vi "CanTest.vi"() -> ()   [LabVIEW 2015]
uses:
  Crl/Can_DataType.ctl
panel:
  in  "SCUBoot":bool
  out "RespGood？":bool
  in  "Clear":bool
  in  "Seq?":bool
  in  "EXIT":bool
  in  "identifier":u32=1238 format="%x"
  in  "select？":bool
  in  "Send Data":T1=[{"identifier"=1715, "payload"=[3, 34, 241, 80, 0, 0, 0, 0], "Send?"=FALSE, "Note"="软件版本", "Delays"=200, "Seq"=0}, {"identifier"=1715, "payload"=[3, 34, 241, 81, 0, 0, 0, 0], "Send?"=FALSE, "Note"="硬件版本", "Delays"=200, "Seq"=0}, {"identifier"=1715, "payload"=[3, 34, 2, 0, 0, 0, 0, 0], "Send?"=FALSE, "Note"="玻璃位置", "Delays"=200, "Seq"=0}, {"identifier"=1715, "payload"=[4, 49, 1, 3, 10, 0, 0, 0], "Send?"=FALSE, "Note"="初始化", "Delays"=200, "Seq"=0}, {"identifier"=1715, "payload"=[5, 49, 1, 3, 2, 2, 0, 0], "Send?"=FALSE, "Note"="玻璃开", "Delays"=200, "Seq"=0}, {"identifier"=1715, "payload"=[4, 46, 254, 17, 4, 0, 0, 0], "Send?"=FALSE, "Note"="设置工厂模式", "Delays"=200, "Seq"=0}] {"payload" format="%02x"; "identifier" format="%x"}
  out "Frames":string[][](table)
  in  "Send":bool
  in  "Number of Frames to Display":i32=1500
  in  "点火":T1=[{"identifier"=1715, "payload"=[2, 16, 3, 255, 255, 255, 255, 255], "Send?"=FALSE, "Note"="", "Delays"=100, "Seq"=0}] {"payload" format="%02x"; "identifier" format="%x"}
  in  "interface":refnum<k21>="CAN2"
  # "ms"
  # "ms"
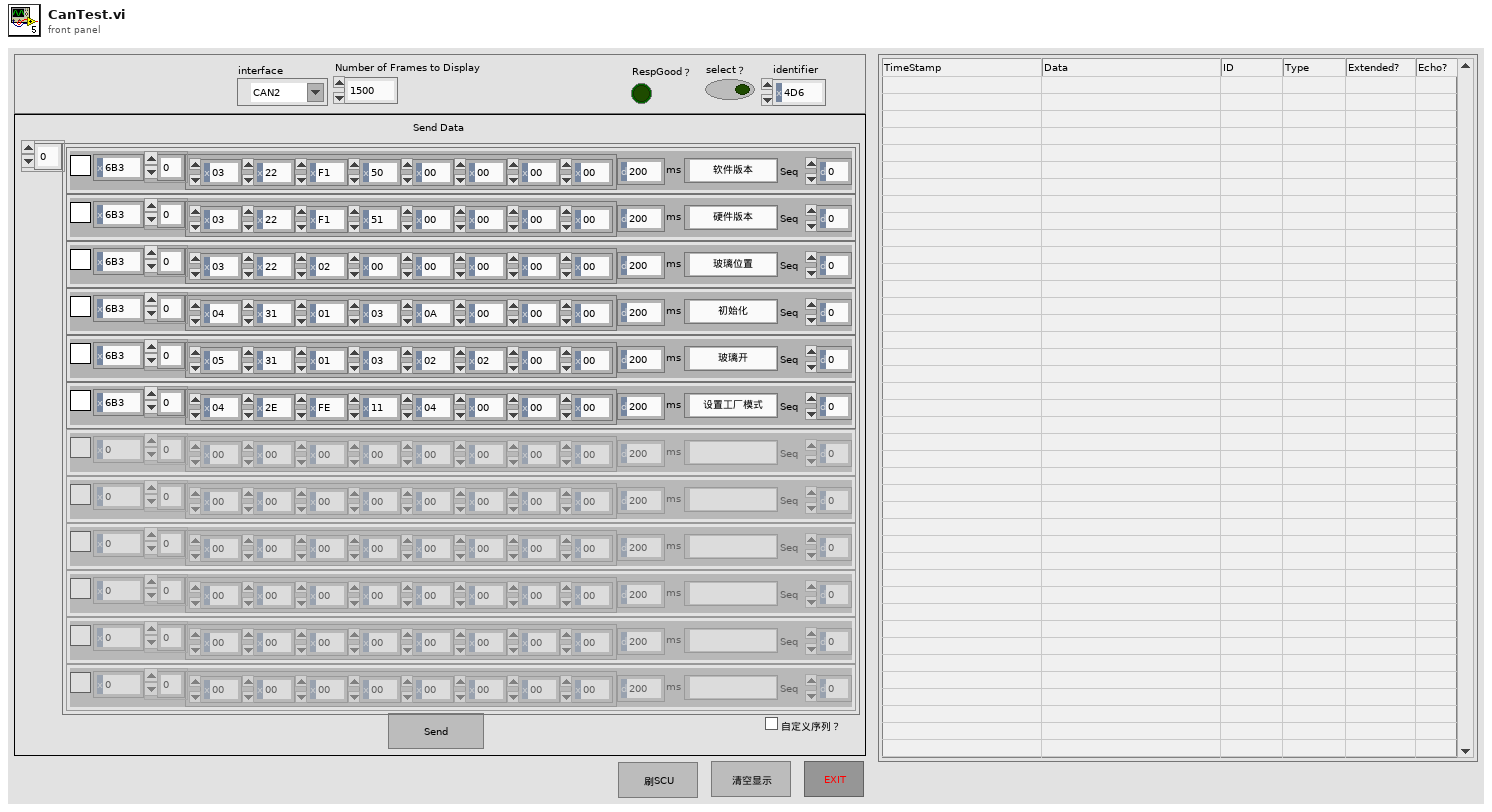
[diagram p1: front panel]
types:
  T1 = typedef "Can_DataType.ctl" = cluster{"identifier":u32, "payload":u8[], "Send?":bool, "Note":string, "Delays":u32, "Seq":i32}[]
  T2 = typedef "XNET Frame CAN.ctl" = cluster{"timestamp":timestamp, "payload":u8[], "identifier":u32, "type":T3, "extended?":bool, "echo?":bool}
  T3 = typedef "XNET Frame Type CAN.ctl" = u8
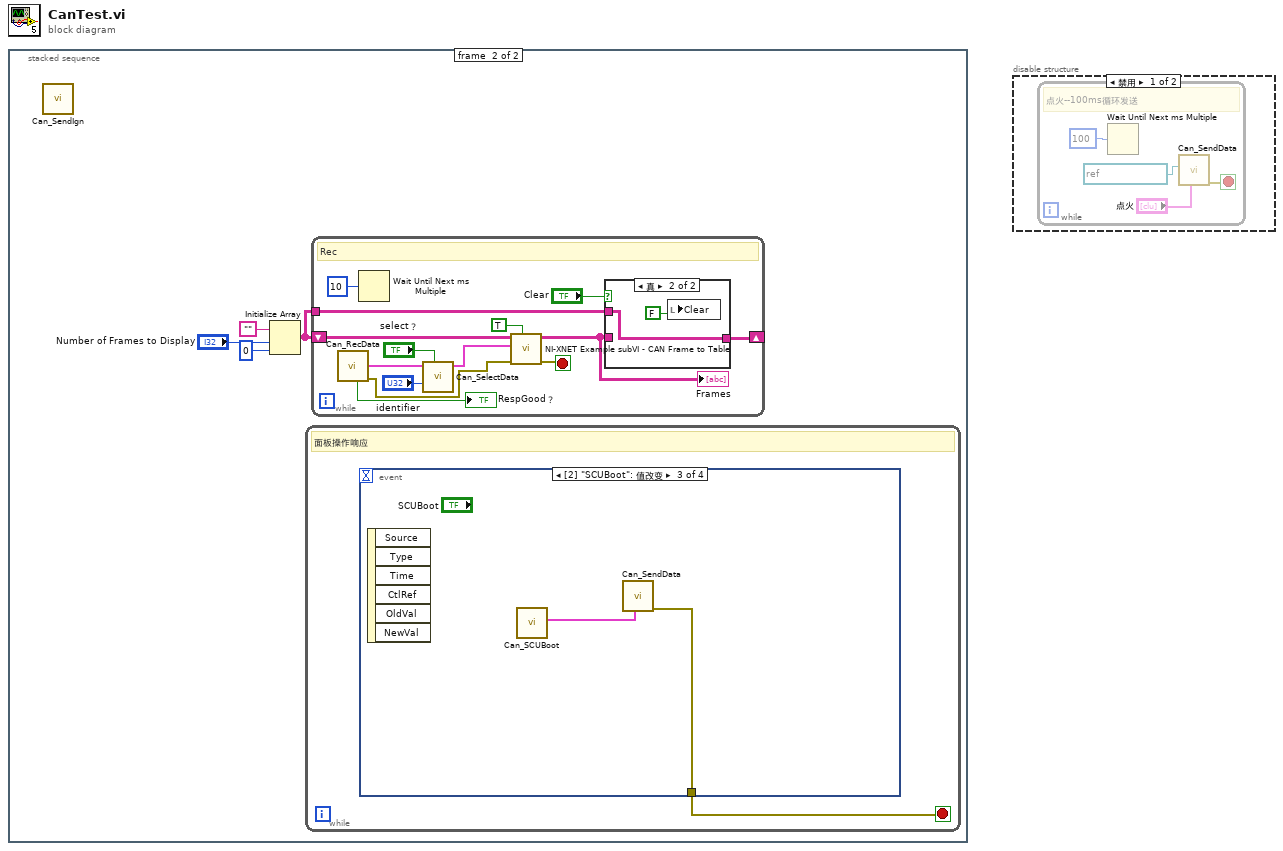
[diagram p0: block diagram]
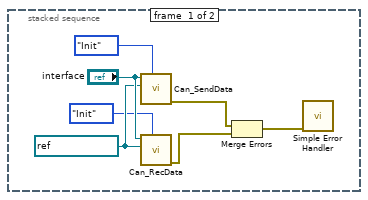
[diagram p3: hidden frame]
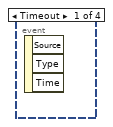
[diagram p4: hidden frame]
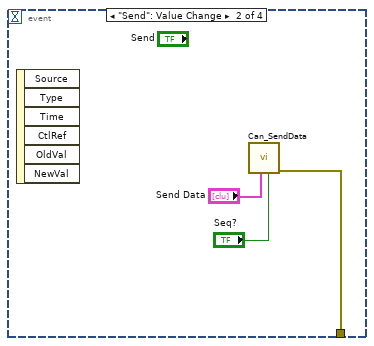
[diagram p5: hidden frame]
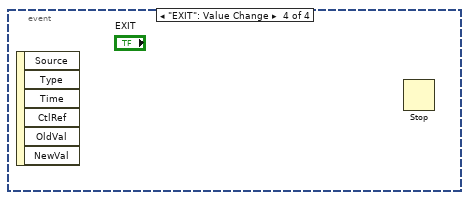
[diagram p6: hidden frame]
diagram:
  n1 = stacked-sequence {
    frame #0 {
      w6 = refnum<k21> "Z177TEST" ("cluster (:memory:)")
      n2 = call "Can_SendData.vi"("mode"=enum16{"Init", "Send"}."Init", "cluster (:memory:)"=w6, "interface"="interface") -> ("error"=w3:errorcluster)  [unwired: 8 in]
      n3 = call "Can_RecData.vi"("mode"=enum16{"Init", "Rec"}."Init", "cluster (:memory:)"=w6, "interface"="interface") -> ("error out"=w2:errorcluster)  [unwired: 6 in, 2 out]
      n4 = Merge Errors(w3, w2) -> (w1:errorcluster)
      n5 = call <vilib>:"Simple Error Handler.vi"("error in (no error)"=w1) -> ()  [unwired: 4 in, 5 out]
    }
    frame #1 {
      n6 = call "Can_SendIgn.vi"() -> ()  [unwired: 12 in]
      n7 = Initialize Array("", "Number of Frames to Display", 0 ("维数大小")) -> (w8:string[][])
      n8 = while {
        stop <- w12 stop-if-true
        # "面板操作响应"
        n9 = event shown="[2] \"SCUBoot\": 值改变" {
          selector: _ -> [_ _ _ _]
          dyn-events: _ -> [_ _ _ _]
          timeout: _ -> [_ _ _ _]
          tunnel: [_ w15 w16 _] -> w12
          event Timeout {
            n10 = event-data() -> ()  [unwired: 1 in, 3 out]
          }
          event "Send": Value Change {
            n11 = event-data() -> ()  [unwired: 1 in, 6 out]
            n12 = call "Can_SendData.vi"("Seq?"="Seq?", "Data"="Send Data") -> ("error"=w15:errorcluster)  [unwired: 9 in]
          }
          event "SCUBoot": Value Change {
            n13 = event-data() -> ()  [unwired: 1 in, 6 out]
            n14 = call "Can_SCUBoot.vi"() -> ("Data"=w17:T1)  [unwired: 11 in]
            n15 = call "Can_SendData.vi"("Data"=w17) -> ("error"=w16:errorcluster)  [unwired: 10 in]
          }
          event "EXIT": Value Change {
            n16 = event-data() -> ()  [unwired: 1 in, 6 out]
            n17 = Stop() -> ()  [unwired: 1 in]
          }
        }
      }
      n18 = while {
        shift-right: [w21] -> _
        shift-left: w8 -> [w29]
        tunnel: w8 -> [w20]
        stop <- w30 stop-if-true
        # "Rec"
        n19 = call "Can_RecData.vi"() -> ("error out"=w18:errorcluster, "data"=w27:T2[], "RespGood？"=→"RespGood？":bool)  [unwired: 9 in]
        n20 = Wait Until Next ms Multiple(millisecond multiple=u32 10 ("milliseconds to wait")) -> ()  [unwired: 1 out]
        n21 = call "Can_SelectData.vi"("select？"="select？", "identifier"="identifier", "data"=w27) -> ("Data"=w26:T2[])  [unwired: 8 in]
        n22 = call "NI-XNET Example subVI - CAN Frame to Table.vi"("Hexadecimal?"=TRUE, "error in (no error)"=w18, "CAN Frames (from XNET Read)"=w26, "Input Array"=w29) -> ("error out"=w30:errorcluster, "Output Array"=w22:string[][])  [unwired: 1 in, 5 out]
        "Frames" <- w22
        n23 = case shown="真" "Clear" {
          tunnel: w22 -> [w32 _]
          tunnel: [w32 w33] -> w21
          tunnel: w20 -> [_ w33]
          frame False {
          }
          frame True {
            n24 = local write "Clear"(FALSE ("Clear")) -> ()
          }
        }
      }
    }
  }
  n25 = disable-structure shown="禁用" {
    frame Disabled {
      n26 = while {
        stop <- w37 stop-if-true
        # "点火--100ms循环发送"
        n27 = Wait Until Next ms Multiple(millisecond multiple=u32 100 ("milliseconds to wait")) -> ()  [unwired: 1 out]
        n28 = call "Can_SendData.vi"("Data"="点火", "cluster (:memory:)"=refnum<k21> "Z177TEST") -> ("error"=w37:errorcluster)  [unwired: 9 in]
      }
    }
    frame Enabled {
    }
  }
